vi "Dump Cum Cnts.vi"(8 "error in":errorcluster, 11 "3010 in":refnum<class "3010.lvclass">) -> (0 "error out":errorcluster, 1 "counts":u32, 2 "time":u32, 3 "3010 out":refnum<class "3010.lvclass">)   [LabVIEW 2012, in "3010.lvclass"]
doc: "Get the number of counts from the CPC since the last time the register was cleared."
uses:
  3010.lvclass
  Controls/CmdStruct.ctl
  Controls/Enum Cmd.ctl
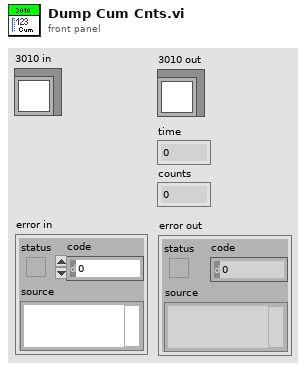
[diagram p1: front panel]
types:
  T1 = typedef "3010.lvclass/Enum Cmd.ctl" = enum16{"Dump", "Dump Cumulative", "Read Liquid Status", "Read Condenser Temperature", "Read Saturator Temperature", "Read Environment", "Read 6 s Buffer", "Read 1 s Buffer", "Read Concentration Display", "Read Delta T", "Read Vacuum Status", "Set Analog Voltage", "Execute Fill", "Clear Display Buffers"}
  T2 = typedef "CmdStruct.ctl" = cluster{"Cmd":u8, "x":i64, "y":i64, "Display":string}
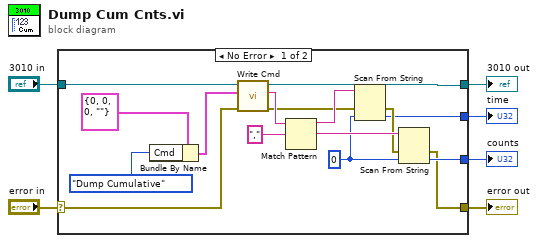
[diagram p0: block diagram]
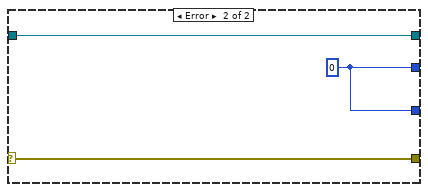
[diagram p2: hidden frame]
diagram:
  n1 = case shown="No Error" "error in" {
    selector: "error in" -> [w20 w25]
    tunnel: [w7 w25] -> w5
    tunnel: [w8 w24] -> w3
    tunnel: "3010 in" -> [w22 w24]
    tunnel: [w10 w23] -> w2
    tunnel: [w9 w23] -> w1
    frame No Error {
      w11 = u32 0 ("default value 1")
      n2 = Bundle By Name(cluster=T2 {"Cmd"=0, "x"=0, "y"=0, "Display"=""} ("CmdStruct"), "Cmd"=Enum_Cmd."Dump Cumulative" ("Enum Cmd")) -> (w18:T2)
      n3 = call-dynamic "Write Cmd.vi"("error in"=w20, "CmdStruct"=w18, "CPC in"=w22) -> ("error out"=w13:errorcluster, "Buffer"=w17:string, "CPC out"=w8:refnum<class "3010.lvclass">)  [unwired: 6 in]
      n4 = Match Pattern(string=w17, regular expression=",") -> (before substring=w14:string, after substring=w15:string)  [unwired: 1 in, 2 out]
      n5 = Scan From String(input string=w14, error in=w13, default 1=w11) -> (error out=w12:errorcluster, output 1=w10:u32)  [unwired: 2 in, 2 out]
      n6 = Scan From String(input string=w15, error in=w12, default 1=w11) -> (error out=w7:errorcluster, output 1=w9:u32)  [unwired: 2 in, 2 out]
    }
    frame Error {
      w23 = u32 0 ("default value 1")
    }
  }
  "error out" <- w5
  "3010 out" <- w3
  "time" <- w2
  "counts" <- w1
